vi "Register.vi"(0 "WAMP Client in":refnum<class "WAMP Client.lvclass">, 1 "Options":string, 5 "Procedure URI":string, 7 "INVOCATION event":refnum<user-event>, 9 "Time Out (ms) (1000)":i32=1000, 11 "error in (no error)":errorcluster) -> (4 "WAMP Client out":refnum<class "WAMP Client.lvclass">, 6 "Success?":bool, 8 "WAMP Error":T1={"Details"="{}", "ArgumentKw Payload"="", "Error?"=FALSE, "Error URI"="", "Arguments Payload"=[]}, 15 "error out":errorcluster)   [LabVIEW 2020, in "wamplv.lvlib" / "WAMP Client.lvclass"]
uses:
  <vilib>/samangh/wamplv/WAMP Client/WAMP Client.lvclass
  <vilib>/samangh/wamplv/WAMP Client/TypeDef/INVOCATION payload.ctl
  <vilib>/samangh/wamplv/WAMP Client/TypeDef/WAMP Error Payload.ctl
  <vilib>/samangh/wamplv/WAMP Client/TypeDef/REGISTERED or ERROR payload.ctl
  <vilib>/samangh/wamplv/WAMP Client/WAMP Client.lvclass/WAMP Client.ctl
  <vilib>/Utility/error.llb/Error Cluster From Error Code.vi
  <vilib>/ErrorRing/Error Ring.xnode
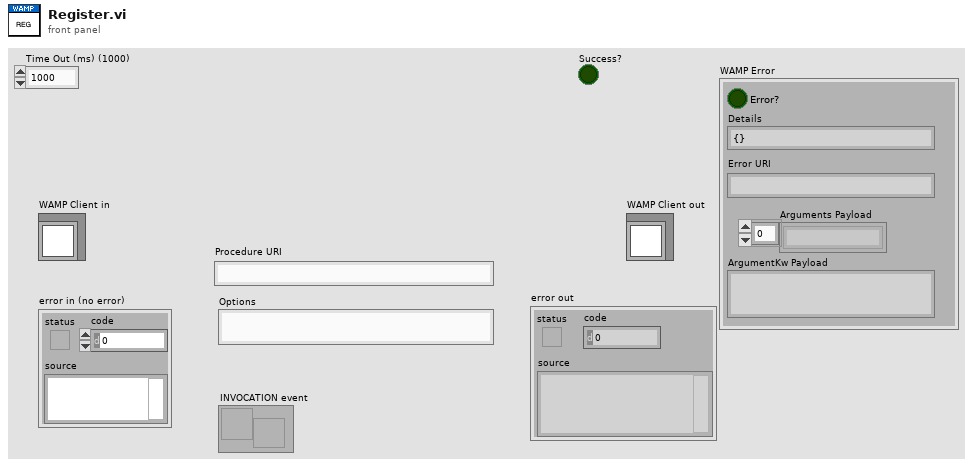
[diagram p1: front panel]
types:
  T1 = typedef "wamplv.lvlib/WAMP Client.lvclass/WAMP Error Payload.ctl" = cluster{"Details":string, "ArgumentKw Payload":string, "Error?":bool, "Error URI":string, "Arguments Payload":string[]}
  T2 = typedef "wamplv.lvlib/WAMP Client.lvclass/REGISTERED or ERROR payload.ctl" = cluster{"Register Request ID":u32, "Registration ID":u32, "Success?":bool, "WAMP Error":T1, "Procedure URI":string}
  T3 = typedef "wamplv.lvlib/WAMP Client.lvclass/Termination Reason.ctl" = cluster{"Reason":T4, "Reason URI":string, "Message":string}
  T4 = typedef "wamplv.lvlib/WAMP Client.lvclass/Termination Reason Enum.ctl" = enum16{"Goodbye Received", "Abort Received", "Send Goodbye", "Send Abort", "Read Loop Failure", "Write Loop Failure", "Message Loop Failure"}
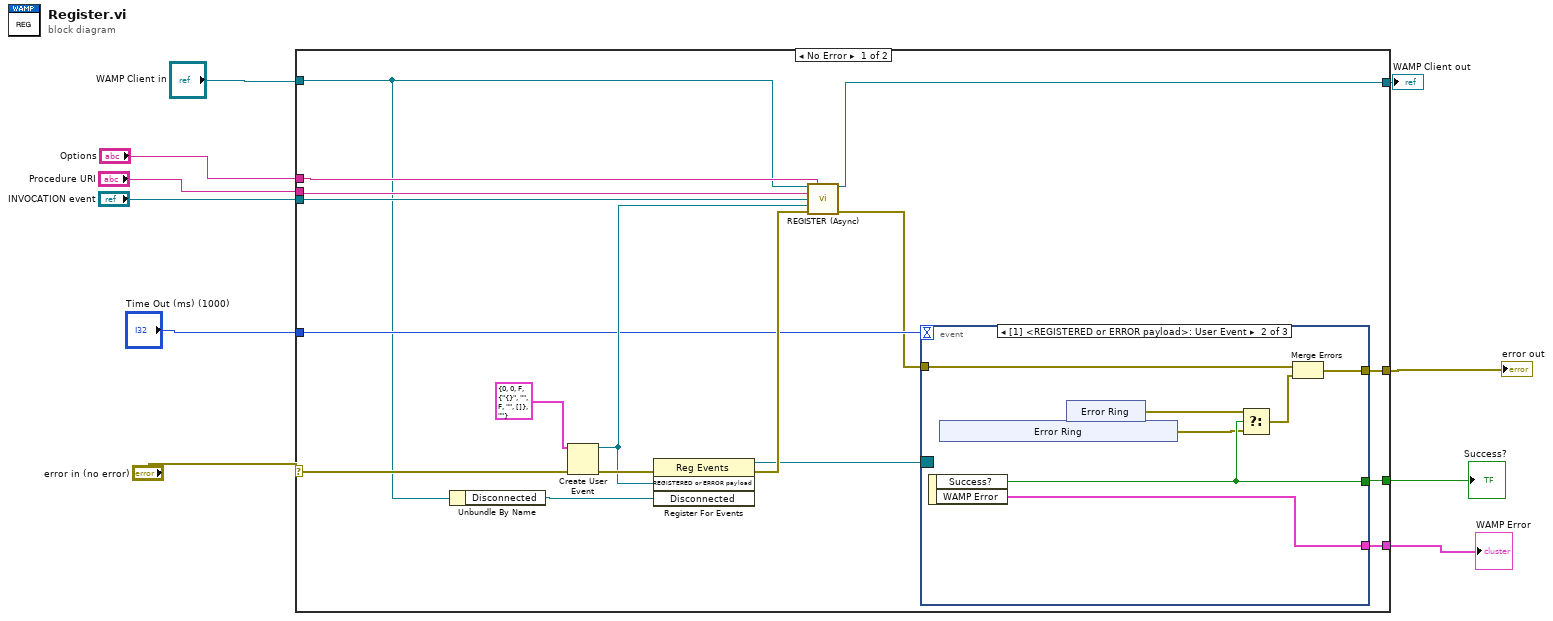
[diagram p0: block diagram]
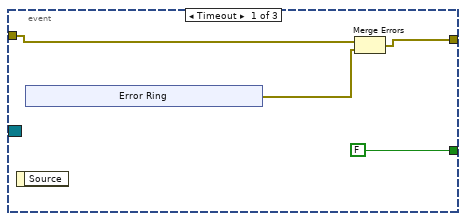
[diagram p2: hidden frame]
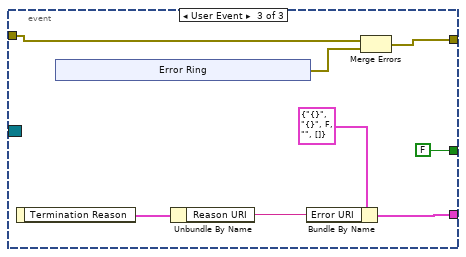
[diagram p3: hidden frame]
diagram:
  n1 = case shown="No Error" "error in (no error)" {
    selector: "error in (no error)" -> [w14 w64]
    tunnel: [w13 w64] -> w1
    tunnel: [w19 w63] -> w8
    tunnel: "WAMP Client in" -> [w12 w63]
    tunnel: "Procedure URI" -> [w27 _]
    tunnel: "Options" -> [w26 _]
    tunnel: "INVOCATION event" -> [w15 _]
    tunnel: "Time Out (ms) (1000)" -> [w20 _]
    tunnel: [w18 _] -> w3
    tunnel: [w17 _] -> w2
    frame No Error {
      n2 = Unbundle By Name(w12) -> ("Disconnected"=w11:refnum<user-event>)
      n3 = Create User Event(user event datatype=T2 {"Register Request ID"=0, "Registration ID"=0, "Success?"=FALSE, "WAMP Error"={"Details"="{}", "ArgumentKw Payload"="", "Error?"=FALSE, "Error URI"="", "Arguments Payload"=[]}, "Procedure URI"=""} ("REGISTERED or ERROR payload"), error in=w14) -> (user event=w23:refnum<user-event>, error out=w24:errorcluster)
      n4 = register-events(error in=w24, w23, w11) -> (reference out=w21:refnum<event-registration>, error out=w22:errorcluster)  [unwired: 1 in]
      n5 = call-dynamic "REGISTER (Async).vi"("WAMP Client in"=w12, "Options"=w26, "Procedure URI"=w27, "INVOCATION event"=w15, "REGISTERED or ERROR event"=w23, "error in (no error)"=w22) -> ("WAMP Client out"=w19:refnum<class "WAMP Client.lvclass">, "error out"=w16:errorcluster)  [unwired: 8 in]
      n6 = event shown="[1] <REGISTERED or ERROR payload>: User Event" {
        selector: w21 -> [_ _ _]
        dyn-events: _ -> [_ _ _]
        timeout: w20 -> [_ _ _]
        tunnel: [FALSE ("Success?") w40 FALSE ("Success?")] -> w18
        tunnel: [_ w43 w53] -> w17
        tunnel: w16 -> [w30 w42 w55]
        tunnel: [w31 w41 w54] -> w13
        event Timeout {
          n7 = event-data() -> ()  [unwired: 1 in, 1 out]
          n8 = xnode "Error Ring"() -> ("error out"=w29:errorcluster)
          n9 = Merge Errors(w30, w29) -> (w31:errorcluster)
        }
        event User Event {
          n10 = event-data() -> ("Success?"=w40:bool, "WAMP Error"=w43:T1)  [unwired: 1 in]
          n11 = xnode "Error Ring"() -> ("error out"=w38:errorcluster)
          n12 = xnode "Error Ring"() -> ("error out"=w39:errorcluster)
          n13 = Select(t=w39, s=w40, f=w38) -> (s? t:f=w37:errorcluster)
          n14 = Merge Errors(w42, w37) -> (w41:errorcluster)
        }
        event User Event {
          n15 = event-data() -> ("Termination Reason"=w51:T3)  [unwired: 1 in]
          n16 = xnode "Error Ring"() -> ("error out"=w57:errorcluster)
          n17 = Unbundle By Name(w51) -> ("Reason URI"=w50:string)
          n18 = Bundle By Name(cluster=T1 {"Details"="{}", "ArgumentKw Payload"="{}", "Error?"=FALSE, "Error URI"="", "Arguments Payload"=[]} ("WAMP Error"), "Error URI"=w50) -> (w53:T1)
          n19 = Merge Errors(w55, w57) -> (w54:errorcluster)
        }
      }
    }
    frame Error {
    }
  }
  "error out" <- w1
  "WAMP Client out" <- w8
  "Success?" <- w3
  "WAMP Error" <- w2
